vi "OP400ZP_Test_DataDyn.vi"(0 "Tcell Min (°C)":dbl, 2 "is30%?":bool, 3 "MCU":bool, 5 "Tcell Max (°C)":dbl, 7 "ISO SPI?":bool, 9 "Température usine (°C)":dbl, 11 "errin":errorcluster, 12 "testname":string="Dyn;", 13 "Vcell Min (V)":dbl, 14 "Vcell Max (V)":dbl) -> (4 "pass":bool, 6 "datalog":string, 8 "Cluster":T1, 10 "StrData":T2, 15 "errout":errorcluster)   [LabVIEW 2020]
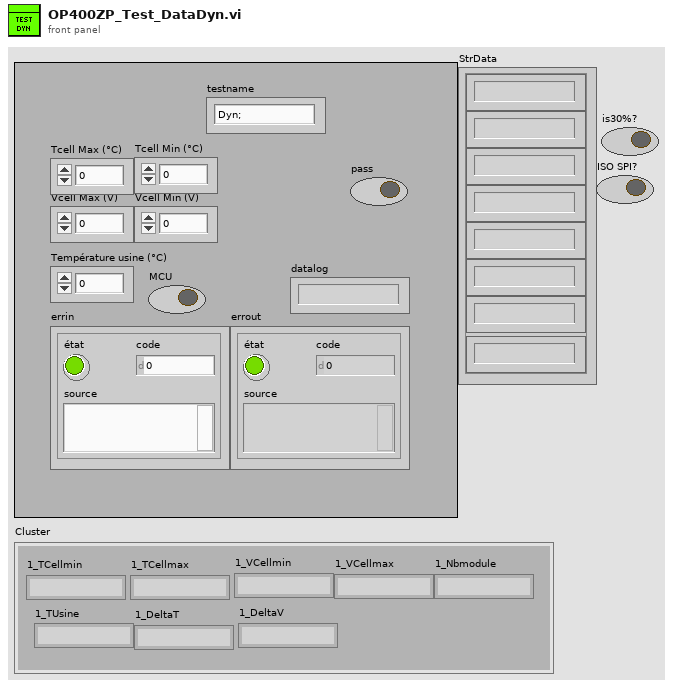
[diagram p1: front panel]
types:
  T1 = cluster{"1_TCellmin":string, "1_TCellmax":string, "1_VCellmin":string, "1_VCellmax":string, "1_Nbmodule":string, "1_TUsine":string, "1_DeltaT":string, "1_DeltaV":string}
  T2 = cluster{"Chaîne":string, "Chaîne":string, "Chaîne":string, "Chaîne":string, "Chaîne":string, "Chaîne":string, "Chaîne":string, "Chaîne 2":string}
  T3 = cluster{string, string, string, string, string, string, string, "cas vrai":string}
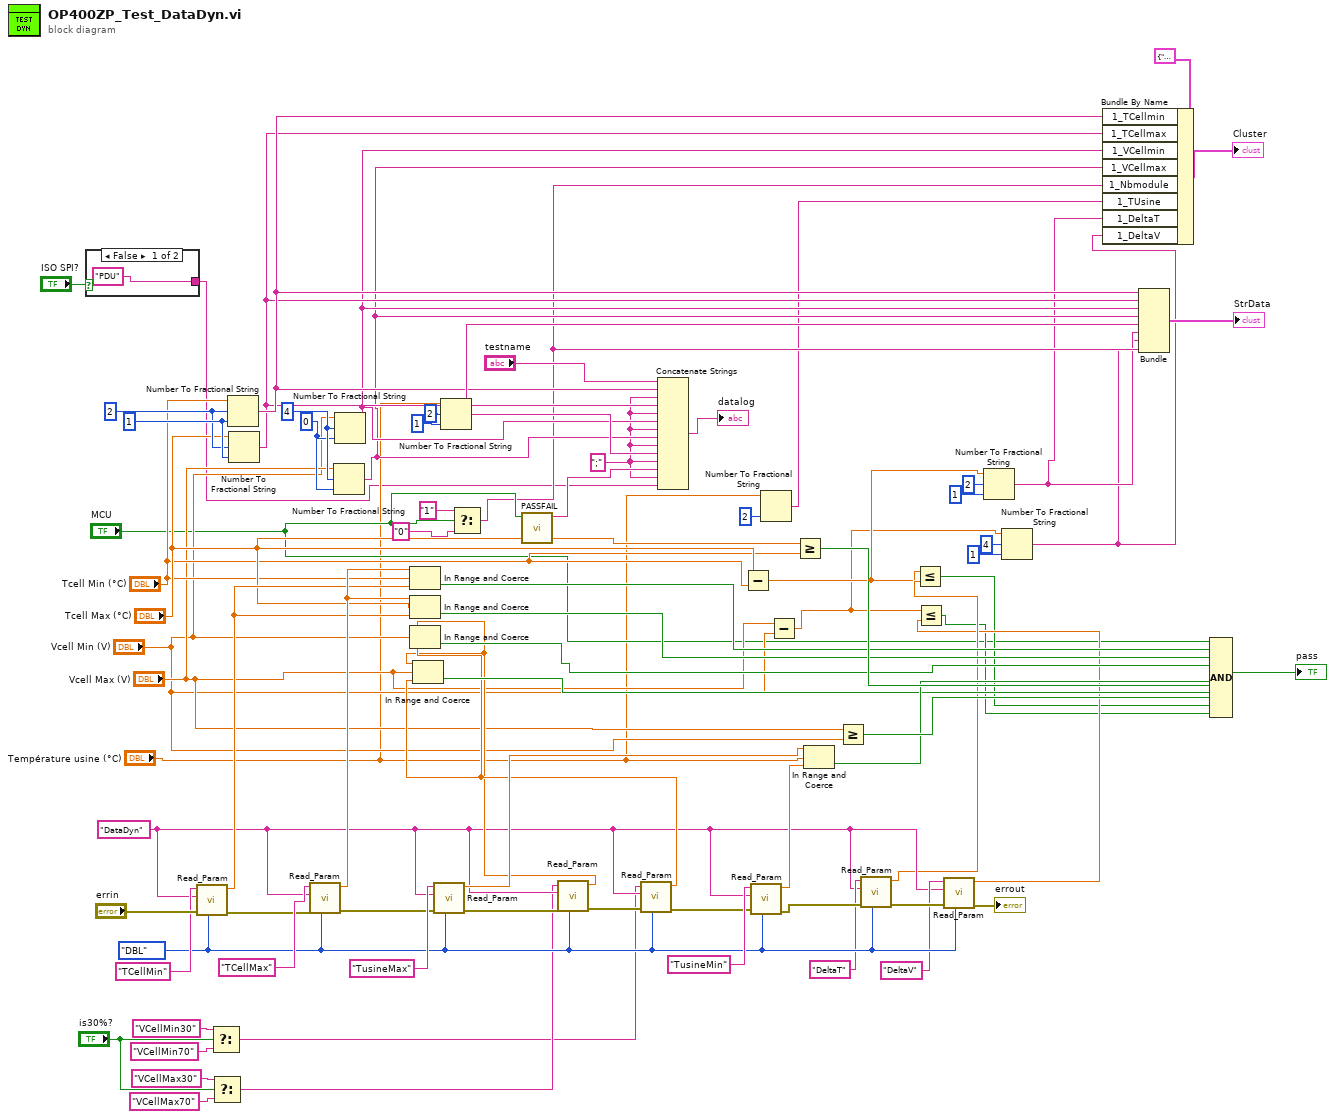
[diagram p0: block diagram]
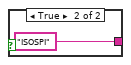
[diagram p2: hidden frame]
diagram:
  w2 = ";" ("chaîne")
  w55 = i16 0 ("précision (6)")
  w56 = i16 4 ("largeur (-)")
  w58 = i16 1 ("précision (6)")
  w57 = i16 2 ("largeur (-)")
  w46 = enum16{"STR", "DBL", "U32"}."DBL" ("Énum")
  w43 = "DataDyn" ("section")
  n1 = case shown="False" "ISO SPI?" {
    tunnel: ["PDU" "ISOSPI"] -> w1
    frame False {
    }
    frame True {
    }
  }
  n2 = call <userlib>:"Read_Param.vi"("Énum"=w46, "errin"="errin", "section"=w43, "key"="TCellMin") -> ("error out"=w59:errorcluster, "dbl"=w65:dbl)  [unwired: 3 in, 3 out]
  n3 = Select ("Sélectionner")(t="VCellMin30" ("key"), s="is30%?", f="VCellMin70" ("key")) -> (s? t:f=w13:string)
  n4 = Select ("Sélectionner")(t="VCellMax30" ("key"), s="is30%?", f="VCellMax70" ("key")) -> (s? t:f=w14:string)
  n5 = Number To Fractional String(number="Tcell Min (°C)", width (-)=w57, precision (6)=w58) -> (F-format string=w24:string)  [unwired: 1 in]
  n6 = Number To Fractional String(number="Tcell Max (°C)", width (-)=w57, precision (6)=w58) -> (F-format string=w23:string)  [unwired: 1 in]
  n7 = call <userlib>:"Read_Param.vi"("Énum"=w46, "errin"=w59, "section"=w43, "key"="TCellMax") -> ("error out"=w60:errorcluster, "dbl"=w67:dbl)  [unwired: 3 in, 3 out]
  n8 = Number To Fractional String(number="Vcell Max (V)", width (-)=w56, precision (6)=w55) -> (F-format string=w21:string)  [unwired: 1 in]
  n9 = Number To Fractional String(number="Vcell Min (V)", width (-)=w56, precision (6)=w55) -> (F-format string=w22:string)  [unwired: 1 in]
  n10 = In Range and Coerce(upper limit=w67, x="Tcell Min (°C)", lower limit=w65) -> (In Range?=w74:bool)  [unwired: 1 out]
  n11 = In Range and Coerce(upper limit=w67, x="Tcell Max (°C)", lower limit=w65) -> (In Range?=w75:bool)  [unwired: 1 out]
  n12 = call <userlib>:"Read_Param.vi"("Énum"=w46, "errin"=w60, "section"=w43, "key"="TusineMax") -> ("error out"=w61:errorcluster, "dbl"=w70:dbl)  [unwired: 3 in, 3 out]
  n13 = Number To Fractional String(number="Température usine (°C)", width (-)=i16 2 ("largeur (-)"), precision (6)=i16 1 ("précision (6)")) -> (F-format string=w50:string)  [unwired: 1 in]
  n14 = Select(t="1" ("cas vrai"), s="MCU", f="0") -> (s? t:f=w20:string)
  n15 = call <userlib>:"PASSFAIL.vi"("E"="MCU") -> ("S"=w26:string)  [unwired: 10 in]
  n16 = call <userlib>:"Read_Param.vi"("Énum"=w46, "errin"=w61, "section"=w43, "key"=w14) -> ("error out"=w62:errorcluster, "dbl"=w68:dbl)  [unwired: 3 in, 3 out]
  n17 = call <userlib>:"Read_Param.vi"("Énum"=w46, "errin"=w62, "section"=w43, "key"=w13) -> ("error out"=w63:errorcluster, "dbl"=w69:dbl)  [unwired: 3 in, 3 out]
  n18 = In Range and Coerce(upper limit=w68, x="Vcell Min (V)", lower limit=w69) -> (In Range?=w76:bool)  [unwired: 1 out]
  n19 = In Range and Coerce(upper limit=w68, x="Vcell Max (V)", lower limit=w69) -> (In Range?=w77:bool)  [unwired: 1 out]
  n20 = Concatenate Strings("testname", w24, w2, w23, w2, w22, w2, w21, w2, w50, w2, w26, w2, w1) -> (→"datalog":string)
  n21 = Subtract(x="Tcell Max (°C)", y="Tcell Min (°C)") -> (x-y=w11:dbl)
  n22 = call <userlib>:"Read_Param.vi"("Énum"=w46, "errin"=w63, "section"=w43, "key"="TusineMin") -> ("error out"=w49:errorcluster, "dbl"=w71:dbl)  [unwired: 3 in, 3 out]
  n23 = Number To Fractional String(number="Température usine (°C)", precision (6)=i16 2 ("précision (6)")) -> (F-format string=w6:string)  [unwired: 2 in]
  n24 = Subtract(x="Vcell Max (V)", y="Vcell Min (V)") -> (x-y=w10:dbl)
  n25 = Greater Or Equal?(x="Tcell Max (°C)", y="Tcell Min (°C)") -> (x >= y?=w79:bool)
  n26 = In Range and Coerce(upper limit=w70, x="Température usine (°C)", lower limit=w71) -> (In Range?=w78:bool)  [unwired: 1 out]
  n27 = Greater Or Equal?(x="Vcell Max (V)", y="Vcell Min (V)") -> (x >= y?=w80:bool)
  n28 = call <userlib>:"Read_Param.vi"("Énum"=w46, "errin"=w49, "section"=w43, "key"="DeltaT") -> ("error out"=w48:errorcluster, "dbl"=w38:dbl)  [unwired: 3 in, 3 out]
  n29 = Less Or Equal?(x=w11, y=w38) -> (x <= y?=w36:bool)
  n30 = call <userlib>:"Read_Param.vi"("Énum"=w46, "errin"=w48, "section"=w43, "key"="DeltaV") -> ("error out"=→"errout":errorcluster, "dbl"=w37:dbl)  [unwired: 3 in, 3 out]
  n31 = Less Or Equal?(x=w10, y=w37) -> (x <= y?=w35:bool)
  n32 = Number To Fractional String(number=w11, width (-)=i16 2 ("largeur (-)"), precision (6)=i16 1 ("précision (6)")) -> (F-format string=w5:string)  [unwired: 1 in]
  n33 = Number To Fractional String(number=w10, width (-)=i16 4 ("largeur (-)"), precision (6)=i16 1 ("précision (6)")) -> (F-format string=w4:string)  [unwired: 1 in]
  n34 = Bundle By Name ("Assembler par nom")(cluster=T1 {"1_TCellmin"="", "1_TCellmax"="", "1_VCellmin"="", "1_VCellmax"="", "1_Nbmodule"="", "1_TUsine"="", "1_DeltaT"="", "1_DeltaV"=""} ("Cluster"), "1_TCellmin"=w24, "1_TCellmax"=w23, "1_VCellmin"=w22, "1_VCellmax"=w21, "1_Nbmodule"=w20, "1_TUsine"=w6, "1_DeltaT"=w5, "1_DeltaV"=w4) -> (→"Cluster":T1)
  n35 = Bundle(w24, w23, w22, w21, w50, w5, w4, "cas vrai"=w20) -> (→"StrData":T3)  [unwired: 1 in]
  n36 = Compound Arithmetic op=AND ("Opérateur arithmétique")("MCU", w74, w75, w76, w77, w78, w79, w80, w36, w35) -> (→"pass":bool)
